vi "AMZ_S3_AUTH_Make HTTP Request v4.vi"(0 "HTTP-Verb":string(combo)="GET", 1 "AWS Service":string="s3", 2 "Region":string="us-east-1", 3 "Bucket":string, 4 "Object Key":string, 5 "error in":errorcluster, 6 "request headers":cluster{"item":string, "value":string}[](array[cluster])=[{"item"="Content-Type", "value"="application/x-amz-json-1.1"}], 7 "request parameters":cluster{"item":string, "value":string}[](array[cluster]), 9 "request body":string) -> (12 "Call Result":T1, 14 "response headers":string, 16 "response body":string, 19 "error out":errorcluster)   [LabVIEW 2015, in "LV Interface for Amazon S3.lvlib"]
uses:
  LV Interface for Amazon S3.lvlib
  Typedefs/AMZ_S3_Call Results.ctl
  <vilib>/regexp/Match Regular Expression.xnode
  <vilib>/httpClient/LabVIEWHTTPClient.lvlib
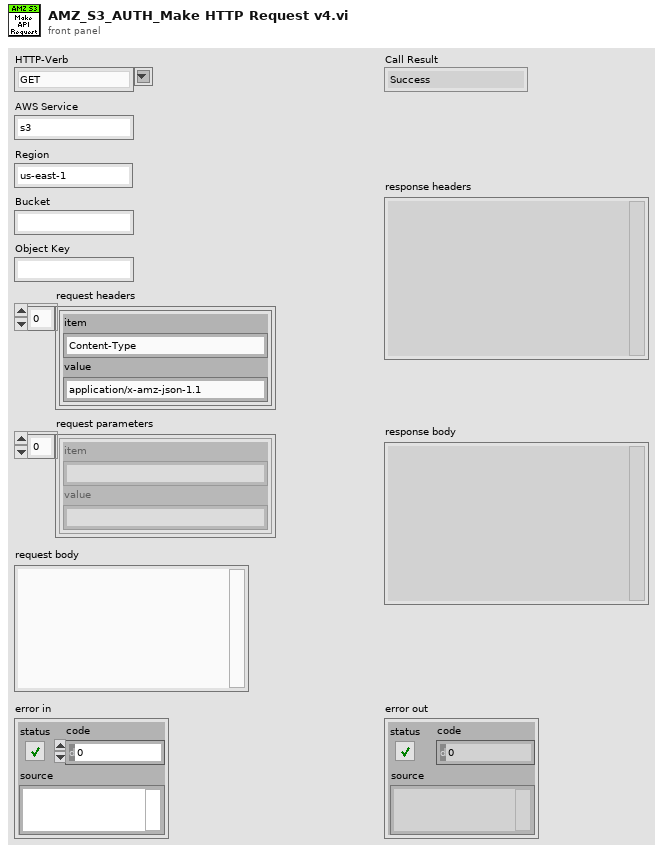
[diagram p1: front panel]
types:
  T1 = typedef "LV Interface for Amazon S3.lvlib/AMZ_S3_Call Results.ctl" = enum16{"Success", "UndefinedError", "AccessDenied", "AccountProblem", "AmbiguousGrantByEmailAddress", "BadDigest", "BucketAlreadyExists", "BucketAlreadyOwnedByYou", "BucketNotEmpty", "CredentialsNotSupported", "CrossLocationLoggingProhibited", "EntityTooSmall", "EntityTooLarge", "ExpiredToken", "IllegalVersioningConfigurationException", "IncompleteBody", "IncorrectNumberOfFilesInPostRequest", "InlineDataTooLarge", "InternalError", "InvalidAccessKeyId", "InvalidAddressingHeader", "InvalidArgument", "InvalidBucketName", "InvalidDigest", "InvalidLocationConstraint", "InvalidPart", "InvalidPartOrder", "InvalidPayer", "InvalidPolicyDocument", "InvalidRange", "InvalidSecurity", "InvalidSOAPRequest", "InvalidStorageClass", "InvalidTargetBucketForLogging", "InvalidToken", "InvalidURI", "KeyTooLong", "MalformedACLError", "MalformedPOSTRequest", "MalformedXML", "MaxMessageLengthExceeded", "MaxPostPreDataLengthExceededError", "MetadataTooLarge", "MethodNotAllowed", "MissingAttachment", "MissingContentLength", "MissingRequestBodyError", "MissingSecurityElement", "MissingSecurityHeader", "NoLoggingStatusForKey", "NoSuchBucket", "NoSuchKey", "NoSuchUpload", "NoSuchVersion", "NotImplemented", "NotSignedUp", "OperationAborted", "PermanentRedirect", "PreconditionFailed", "Redirect", "RequestIsNotMultiPartContent", "RequestTimeout", "RequestTimeTooSkewed", "RequestTorrentOfBucketError", "SignatureDoesNotMatch", "SlowDown", "TemporaryRedirect", "TokenRefreshRequired", "TooManyBuckets", "UnexpectedContent", "UnresolvableGrantByEmailAddress", "UserKeyMustBeSpecified", "LabVIEWError"}
  T2 = typedef "LabVIEWHTTPClient.lvlib/ClientHandle.ctl" = refnum<k1>
  T3 = typedef "LV Interface for Amazon S3.lvlib/AMZ_S3_AWS Credentials.ctl" = cluster{"Access Key":string, "Secret Key":string}
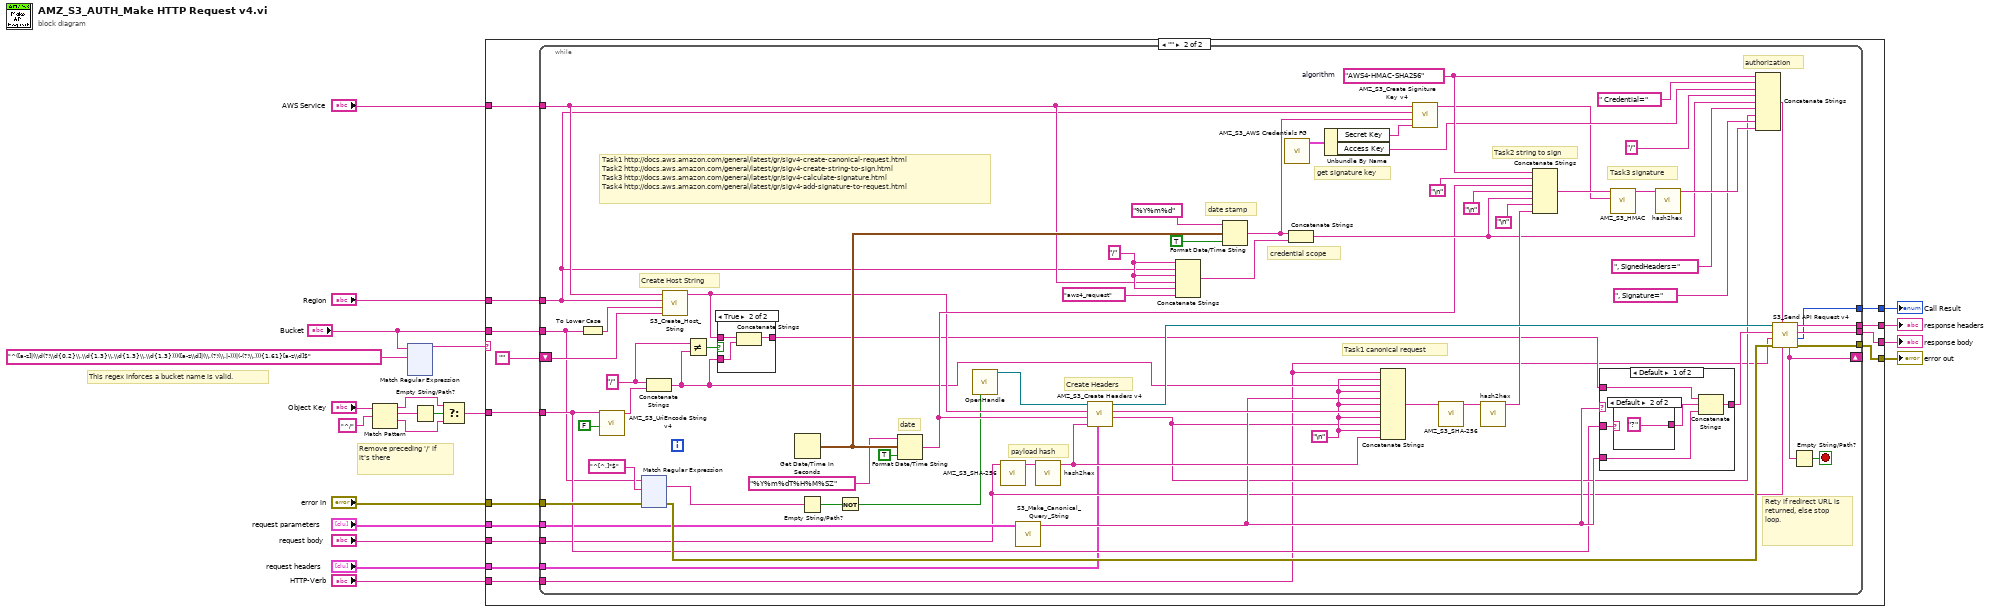
[diagram p0: block diagram]
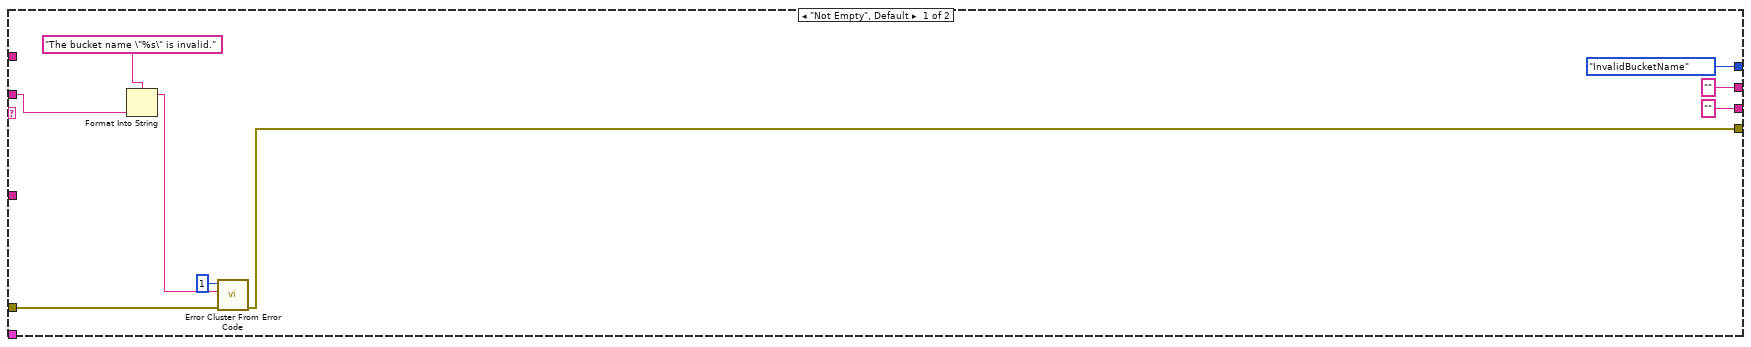
[diagram p2: hidden frame]
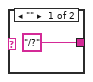
[diagram p4: hidden frame]
diagram:
  # "This regex inforces a bucket name is valid."
  # "Remove preceding '/' if it's there"
  n1 = Match Pattern(string="Object Key", regular expression="^/") -> (before substring=w15:string, match substring=w13:string, after substring=w16:string)  [unwired: 1 in, 1 out]
  n2 = xnode "Match Regular Expression"("input string"="Bucket", "regular expression"="^([a-z]|(\\d(?!\\d{0,2}\\.\\d{1,3}\\.\\d{1,3}\\.\\d{1,3})))([a-z\\d]|(\\.(?!(\\.|-)))|(-(?!\\.))){1,61}[a-z\\d]$") -> ("before match"=w3:string)  [unwired: 4 in, 4 out]
  n3 = Empty String/Path?(string/path=w13) -> (empty?=w14:bool)
  n4 = Select(t=w15, s=w14, f=w16) -> (s? t:f=w11:string)
  n5 = case shown="\"\"" w3 {
    tunnel: ["" ("response headers") w44] -> w21
    tunnel: [AMZ_S3_Call_Results."InvalidBucketName" ("Call Result") w43] -> w20
    tunnel: [w25 w42] -> w19
    tunnel: ["" ("response body") w41] -> w18
    tunnel: "error in" -> [w28 w40]
    tunnel: w11 -> [_ w39]
    tunnel: "AWS Service" -> [_ w38]
    tunnel: "Region" -> [_ w37]
    tunnel: "Bucket" -> [w30 w36]
    tunnel: "request parameters" -> [_ w35]
    tunnel: "request body" -> [_ w34]
    tunnel: "request headers" -> [_ w33]
    tunnel: "HTTP-Verb" -> [_ w32]
    frame "Not Empty", Default {
      n6 = Format Into String(format string="The bucket name \"%s\" is invalid.", w30) -> (resulting string=w27:string)  [unwired: 2 in, 1 out]
      n7 = call <vilib>:"Error Cluster From Error Code.vi"("error in (no error)"=w28, "error message (\"\")"=w27, "error code (0)"=1) -> ("error out"=w25:errorcluster)  [unwired: 6 in]
    }
    frame "" {
      n8 = while {
        tunnel: [w112] -> w44
        tunnel: [w64] -> w42
        tunnel: [w69] -> w41
        shift-right: [w68] -> _
        shift-left: "" ("Redirect endpoint") -> [w66]
        tunnel: [w65] -> w43
        tunnel: w40 -> [w56]
        tunnel: w39 -> [w52]
        tunnel: w38 -> [w51]
        tunnel: w37 -> [w50]
        tunnel: w36 -> [w49]
        tunnel: w35 -> [w48]
        tunnel: w34 -> [w47]
        tunnel: w33 -> [w46]
        tunnel: w32 -> [w45]
        stop <- w67 stop-if-true
        w74 = "/" ("string")
        w86 = "/" ("string")
        w104 = "AWS4-HMAC-SHA256"  # algorithm
        w81 = "\n"
        # "Rety if redirect URL is returned, else stop loop."
        # "Create Host String"
        # "Task1 canonical request"
        # "Create Headers"
        # "get signature key"
        # "Task1 http://docs.aws.amazon.com/general/latest/gr/sigv4-create-canonical-request.html\nTask2 http://docs.aws.amazon.com/general/latest/gr/sigv4-create-string-to-sign.html\nTask3 http://docs.aws.amazon.com/general/latest/gr/sigv4-calculate-signature.html\nTask4 http://docs.aws.amazon.com/general/latest/gr/sigv4-add-signature-to-request.html"
        # "date stamp"
        # "date"
        # "payload hash"
        # "authorization"
        # "Task3 signature"
        # "Task2 string to sign"
        # "credential scope"
        n9 = To Lower Case(string=w49) -> (all lower case string=w62:string)
        n10 = call "AMZ_S3_UriEncode String v4.vi"("Encode /"=FALSE, "Un-encoded String"=w52) -> ("UriEncoded String"=w54:string)  [unwired: 9 in]
        n11 = xnode "Match Regular Expression"("input string"=w49, "regular expression"="^[^.]*$", "error in"=w56) -> ("whole match"=w60:string, "error out"=w57:errorcluster)  [unwired: 3 in, 3 out]
        n12 = Concatenate Strings(w74, w54) -> (w71:string)
        n13 = call "S3_Create_Host_String.vi"("Redirect Endpoint"=w66, "Bucket"=w62, "Region"=w50, "AWS Service"=w51) -> ("Host String"=w72:string)  [unwired: 7 in]
        n14 = Not Equal?(x=w74, y=w71) -> (x != y?=w73:bool)
        n15 = case shown="True" w73 {
          tunnel: w72 -> [w227 w230]
          tunnel: w71 -> [_ w229]
          tunnel: [w227 w228] -> w70
          frame False {
          }
          frame True {
            n16 = Concatenate Strings(w230, w229) -> (w228:string)
          }
        }
        n17 = Get Date/Time In Seconds() -> (seconds since 1Jan1904=w78:timestamp)
        n18 = Empty String/Path?(string/path=w60) -> (empty?=w59:bool)
        n19 = Not(x=w59) -> (.not. x?=w58:bool)
        n20 = Format Date/Time String(time format string (%c)="%Y%m%dT%H%M%SZ", seconds (now)=w78, UTC format=TRUE) -> (date/time string=w79:string)
        n21 = call <vilib>:"OpenHandle.vi"("verify server(true)"=w58) -> ("client handle out"=w82:T2)  [unwired: 13 in, 1 out]
        n22 = call "AMZ_S3_SHA-256.vi"("Message"=w47) -> ("Hash Value"=w96:string)  [unwired: 10 in]
        n23 = call "S3_Make_Canonical_Query_String.vi"("request parameters"=w48) -> ("canonical parameters"=w75:string)  [unwired: 10 in]
        n24 = call "hash2hex.vi"("hash string"=w96) -> ("hex string"=w80:string)  [unwired: 10 in]
        n25 = call "AMZ_S3_Create Headers v4.vi"("request headers"=w46, "RequestBody Payload"=w80, "date/time string"=w79, "Host"=w72, "Client Handle In"=w82) -> ("Signed Headers"=w63:string, "canonical headers"=w100:string, "Client Handle Out"=w110:T2)  [unwired: 3 in]
        n26 = Concatenate Strings(w86, w50, w86, w51, w86, "aws4_request" ("string")) -> (w87:string)
        n27 = Format Date/Time String(time format string (%c)="%Y%m%d", seconds (now)=w78, UTC format=TRUE) -> (date/time string=w93:string)
        n28 = call "AMZ_S3_AWS Credentials FG.vi"() -> ("AWS Credentials"=w84:T3)  [unwired: 10 in, 1 out]
        n29 = Concatenate Strings(w93, w87) -> (w88:string)
        n30 = Unbundle By Name(w84) -> ("Secret Key"=w83:string, "Access Key"=w90:string)
        n31 = Concatenate Strings(w45, w81, w71, w81, w75, w81, w100, w81, w63, w81, w80) -> (w95:string)
        n32 = call "AMZ_S3_Create Signiture Key v4.vi"("AWS Service"=w51, "Region"=w50, "date/time string"=w93, "Secret Key"=w83) -> ("Keyed-Hash"=w55:string)  [unwired: 6 in]
        n33 = call "AMZ_S3_SHA-256.vi"("Message"=w95) -> ("Hash Value"=w94:string)  [unwired: 10 in]
        n34 = call "hash2hex.vi"("hash string"=w94) -> ("hex string"=w103:string)  [unwired: 10 in]
        n35 = Concatenate Strings(w104, "\n", w79, "\n", w88, "\n", w103) -> (w92:string)
        n36 = case shown="Default" w75 {
          tunnel: [w235 w238] -> w76
          tunnel: w70 -> [w233 w238]
          tunnel: w75 -> [w234 _]
          tunnel: w52 -> [w231 _]
          frame Default {
            n37 = case shown="Default" w231 {
              tunnel: ["/?" ("string") "?" ("string")] -> w232
              frame "" {
              }
              frame Default {
              }
            }
            n38 = Concatenate Strings(w233, w232, w234) -> (w235:string)
          }
          frame "" {
          }
        }
        n39 = call "AMZ_S3_HMAC.vi"("Key"=w55, "Message"=w92) -> ("Keyed Hash"=w91:string)  [unwired: 9 in]
        n40 = call "hash2hex.vi"("hash string"=w91) -> ("hex string"=w109:string)  [unwired: 10 in]
        n41 = Concatenate Strings(w104, " Credential=", w90, "/", w88, ", SignedHeaders=", w63, ", Signature=", w109) -> (w111:string)
        n42 = call "S3_Send API Request v4.vi"("request body"=w47, "Authorization"=w111, "error in (no error)"=w57, "HTTP-Verb"=w45, "Host String"=w76, "Client Handle In"=w110) -> ("error out"=w64:errorcluster, "Call Result"=w65:T1, "response body"=w69:string, "response headers"=w112:string, "Redirect endpoint"=w68:string)  [unwired: 1 in]
        n43 = Empty String/Path?(string/path=w68) -> (empty?=w67:bool)
      }
    }
  }
  "response headers" <- w21
  "response body" <- w18
  "error out" <- w19
  "Call Result" <- w20
